vi "shuttersCloseShutter.vi"(1 "shutter":i32) -> ()   [LabVIEW 2017]
uses:
  globalDevices.vi
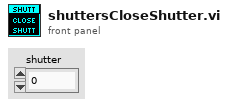
[diagram p1: front panel]
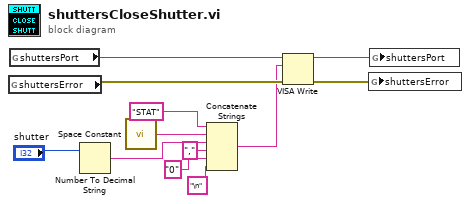
[diagram p0: block diagram]
diagram:
  n1 = global read "globalDevices.vi" "shuttersError"() -> (w11:errorcluster)
  n2 = global read "globalDevices.vi" "shuttersPort"() -> (w12:refnum<visa-resource-name>)
  n3 = Number To Decimal String(number="shutter") -> (decimal integer string=w7:string)  [unwired: 1 in]
  n4 = call <vilib>:"Space Constant.vi"() -> ("String"=w8:string)
  n5 = Concatenate Strings("STAT", w8, w7, "," ("string"), "0" ("string"), "\n" ("string")) -> (w4:string)
  n6 = VISA Write(VISA resource name=w12, write buffer=w4, error in (no error)=w11) -> (VISA resource name out=w3:refnum<visa-resource-name>, error out=w2:errorcluster)  [unwired: 1 out]
  n7 = global write "globalDevices.vi" "shuttersError"(w2) -> ()
  n8 = global write "globalDevices.vi" "shuttersPort"(w3) -> ()
